vi "Signalverlaeufe in Graphen Umladen mit Refernzwert.vi"(4 "Deviation":sgl[](array[numeric]), 6 "Mittelwertdaten":sgl[][](array[numeric]), 8 "Gas-Auswahl":T1, 9 "t0":timestamp, 10 "Referenz in":sgl, 11 "Werte":sgl[][](array[numeric])) -> (0 "Konzentration":sgl, 1 "Refernz":waveform(sgl) caption="Referenz (Ausgang)", 2 "Mittelwert":waveform(dbl), 3 "Waveform":waveform(dbl), 5 "aktuelle Mittelwert":sgl, 7 "Deviation":sgl)   [LabVIEW 2020, in "EPA 1065.lvlib" / "HovaCAL Interference verificaton.lvlib"]
uses:
  HovaCAL Interference verificaton.lvlib
  Visualisierungs Elemente/Auswahlfeld.ctl
  Seiten/FT-IR/FGV FT-IR Aktionen.ctl
  Seiten/FT-IR/FT-IR.lvlib
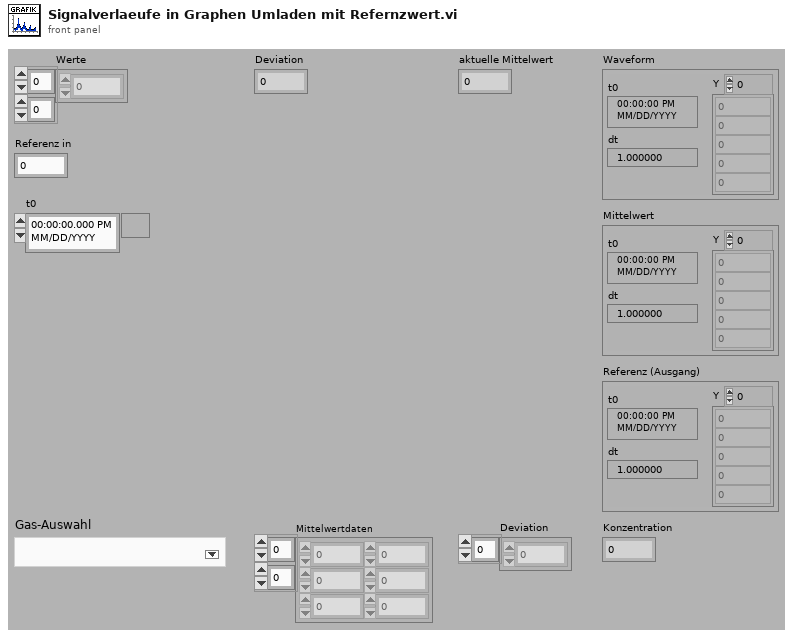
[diagram p1: front panel]
types:
  T1 = typedef "Auswahlfeld.ctl" = u16
  T2 = typedef "FT-IR.lvlib/FGV FT-IR Aktionen.ctl" = enum16{"lesen", "NOG setzen", "NOS setzen", "Initialisieren", "speichern", "ALLES setzen", "FT-IR Spektrum loggen", "Komm Stoppen", "Spektrum LogKonfig"}
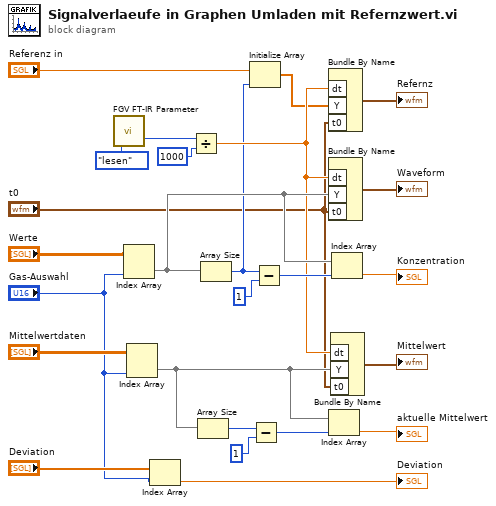
[diagram p0: block diagram]
diagram:
  n1 = call "FGV FT-IR Parameter.vi"("Aktion"=FGV_FT-IR_Aktionen."lesen") -> ("Zykluszeit Messdatenverteiler"=w9:u32)  [unwired: 11 in, 7 out]
  n2 = Index Array(array="Werte", index (col)="Gas-Auswahl") -> (element=w20:sgl[])  [unwired: 1 in]
  n3 = Index Array(array="Mittelwertdaten", index (col)="Gas-Auswahl") -> (element=w13:sgl[])  [unwired: 1 in]
  n4 = Index Array(array="Deviation", index="Gas-Auswahl") -> (element=→"Deviation":sgl)
  n5 = Divide(x=w9, y=u32 1000) -> (x/y=w6:dbl)
  n6 = Array Size(array=w13) -> (size(s)=w15:i32)
  n7 = Array Size(array=w20) -> (size(s)=w5:i32)
  n8 = Initialize Array("Referenz in", w5) -> (w3:sgl[])
  n9 = Subtract(x=w15, y=1) -> (x-y=w17:i32)
  n10 = Subtract(x=w5, y=1) -> (x-y=w23:i32)
  n11 = Bundle By Name("dt"=w6, "Y"=w3, "t0"="t0") -> (→"Refernz":waveform(sgl))  [unwired: 1 out]
  n12 = Bundle By Name("dt"=w6, "Y"=w20, "t0"="t0") -> (→"Waveform":waveform(sgl))  [unwired: 1 out]
  n13 = Index Array(array=w13, index=w17) -> (element=→"aktuelle Mittelwert":sgl)
  n14 = Bundle By Name("dt"=w6, "Y"=w13, "t0"="t0") -> (→"Mittelwert":waveform(sgl))  [unwired: 1 out]
  n15 = Index Array(array=w20, index=w23) -> (element=→"Konzentration":sgl)
